vi "HandWashingMachine.vi"() -> ()   [LabVIEW 2020]
uses:
  <vilib>/Instr/_visa.llb/VISA Configure Serial Port (Instr).vi
panel:
  out "bien tro":dbl
  out "Dial":dbl(knob) scale=0.0..255.0
  in  "Water Pump":bool
  in  "Fan":bool
  in  "VISA resource name":refnum<visa-resource-name>
  out "?":dbl(graph)
  out "HCSR04 Sensor":dbl
  out "IR Sensor":dbl
  out "IR":bool
  # "May say va rua tay tu dong"
  # "HCSR04 Sensor"
  # "IR Sensor"
  # "Resistor"
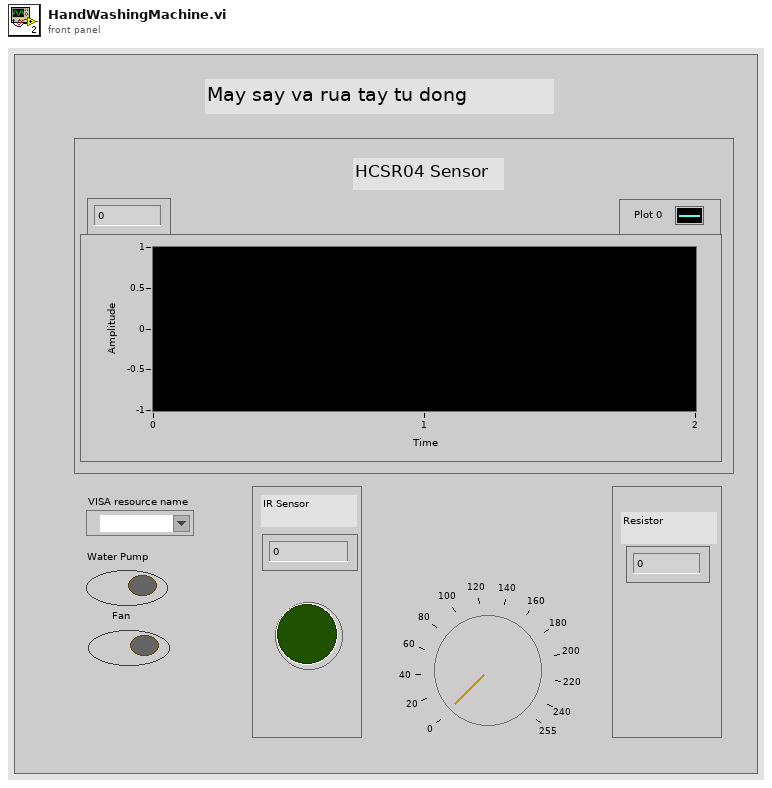
[diagram p1: front panel]
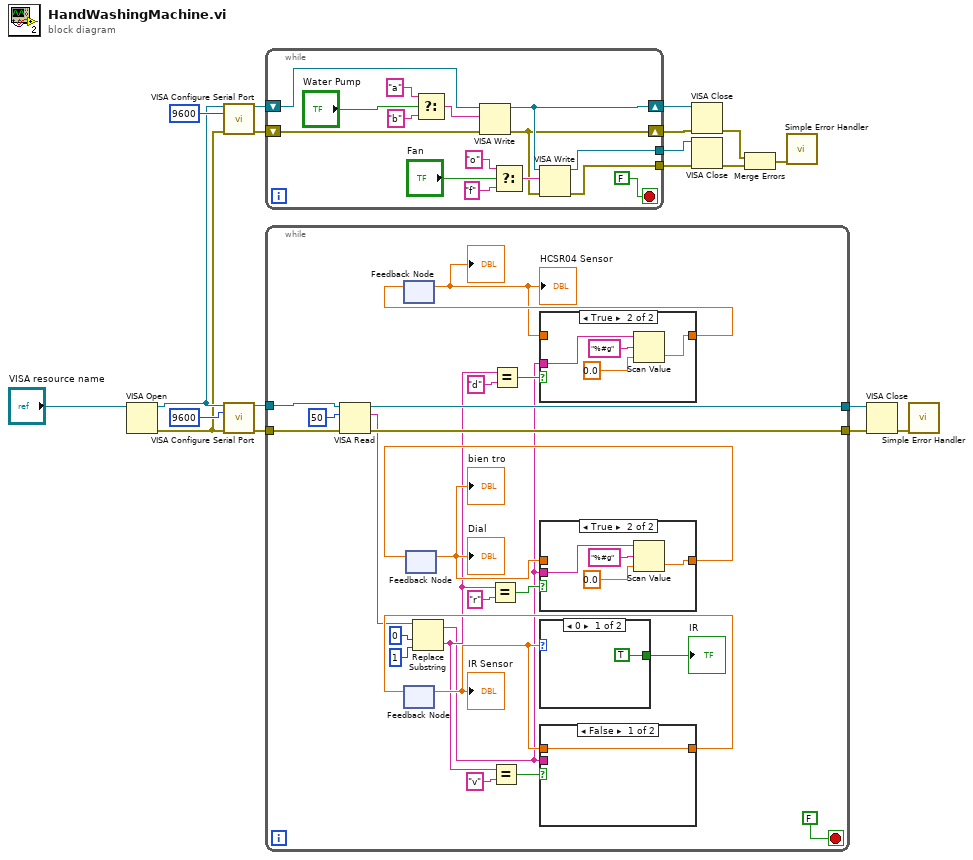
[diagram p0: block diagram]
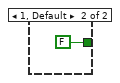
[diagram p3: hidden frame]
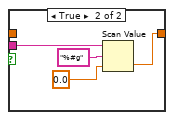
[diagram p4: hidden frame]
diagram:
  n1 = VISA Open(VISA resource name="VISA resource name") -> (VISA resource name=w4:refnum<visa-resource-name>, error out=w3:errorcluster)  [unwired: 4 in]
  n2 = call-poly "VISA Configure Serial Port"("VISA resource name"=w4, "baud rate (9600)"=u32 9600, "error in (no error)"=w3) -> ("VISA resource name out"=w2:refnum<visa-resource-name>, "error out"=w1:errorcluster)  [unwired: 11 in]
  n3 = call-poly "VISA Configure Serial Port"("VISA resource name"=w4, "baud rate (9600)"=u32 9600, "error in (no error)"=w3) -> ("VISA resource name out"=w19:refnum<visa-resource-name>, "error out"=w18:errorcluster)  [unwired: 11 in]
  n4 = while {
    shift-right: [w21] -> w10
    shift-left: w2 -> [w22]
    shift-right: [w20] -> w9
    shift-left: w1 -> [w28]
    tunnel: [w31] -> w12
    tunnel: [w30] -> w11
    stop <- FALSE stop-if-true
    n5 = Select(t="a", s="Water Pump", f="b") -> (s? t:f=w32:string)
    n6 = VISA Write(VISA resource name=w22, write buffer=w32, error in (no error)=w28) -> (VISA resource name out=w21:refnum<visa-resource-name>, error out=w20:errorcluster)  [unwired: 1 out]
    n7 = Select(t="o", s="Fan", f="f") -> (s? t:f=w23:string)
    n8 = VISA Write(VISA resource name=w21, write buffer=w23, error in (no error)=w20) -> (VISA resource name out=w31:refnum<visa-resource-name>, error out=w30:errorcluster)  [unwired: 1 out]
  }
  n9 = while {
    tunnel: w19 -> [w42]
    tunnel: [w56] -> w17
    tunnel: w18 -> [w41]
    tunnel: [w55] -> w16
    stop <- FALSE stop-if-true
    n10 = VISA Read(VISA resource name=w42, byte count=u32 50, error in (no error)=w41) -> (VISA resource name out=w56:refnum<visa-resource-name>, read buffer=w43:string, error out=w55:errorcluster)  [unwired: 1 out]
    n11 = feedback #1() -> (w51:dbl)  [unwired: 1 in]
    "HCSR04 Sensor" <- w51
    "?" <- w51
    n12 = feedback #2() -> (w46:dbl)  [unwired: 1 in]
    "IR Sensor" <- w46
    n13 = feedback #3() -> (w37:dbl)  [unwired: 1 in]
    "bien tro" <- w37
    "Dial" <- w37
    n14 = Replace Substring(2:1 ("length (len. of substring)"), 3:0 ("offset (0)"), 5:w43) -> (0:w36:string, 1:w35:string)  [unwired: 1 in]
    n15 = Equal?(x=w36, y="r") -> (x = y?=w39:bool)
    n16 = Equal?(x=w36, y="v") -> (x = y?=w49:bool)
    n17 = Equal?(x=w36, y="d") -> (x = y?=w53:bool)
    n18 = case shown="True" w53 {
      tunnel: w35 -> [_ w74]
      tunnel: [w71 w73] -> w52
      tunnel: w51 -> [w71 _]
      frame False {
      }
      frame True {
        n19 = Scan Value(string=w74, format string="%#g", default (0 dbl)=0.0) -> (value=w73:dbl)  [unwired: 1 out]
      }
    }
    n20 = feedback-in #1(w52) -> ()
    n21 = case shown="True" w39 {
      tunnel: w35 -> [_ w62]
      tunnel: [w59 w61] -> w38
      tunnel: w37 -> [w59 _]
      frame False {
      }
      frame True {
        n22 = Scan Value(string=w62, format string="%#g", default (0 dbl)=0.0) -> (value=w61:dbl)  [unwired: 1 out]
      }
    }
    n23 = feedback-in #3(w38) -> ()
    n24 = case shown="0" w46 {
      tunnel: [TRUE ("IR Sensor") FALSE ("IR Sensor")] -> w47
      frame 0 {
      }
      frame 1, Default {
      }
    }
    "IR" <- w47
    n25 = case shown="False" w49 {
      tunnel: w35 -> [_ w69]
      tunnel: [w66 w68] -> w48
      tunnel: w46 -> [w66 _]
      frame False {
      }
      frame True {
        n26 = Scan Value(string=w69, format string="%#g", default (0 dbl)=0.0) -> (value=w68:dbl)  [unwired: 1 out]
      }
    }
    n27 = feedback-in #2(w48) -> ()
  }
  n28 = VISA Close(VISA resource name=w10, error in (no error)=w9) -> (error out=w7:errorcluster)
  n29 = VISA Close(VISA resource name=w12, error in (no error)=w11) -> (error out=w6:errorcluster)
  n30 = Merge Errors(w7, w6) -> (w5:errorcluster)
  n31 = call <vilib>:"Simple Error Handler.vi"("error in (no error)"=w5) -> ()  [unwired: 4 in, 5 out]
  n32 = VISA Close(VISA resource name=w17, error in (no error)=w16) -> (error out=w14:errorcluster)
  n33 = call <vilib>:"Simple Error Handler.vi"("error in (no error)"=w14) -> ()  [unwired: 4 in, 5 out]
